vi "TS Calibrate Zero.vi"(8 "error out":errorcluster, 11 "GPIB as string":string="6") -> (0 "error out 2":errorcluster, 3 "GPIB # (out)":string)   [LabVIEW 2015]
uses:
  mc2mc4.llb/MC2/MC4 Wait&ParseSRQ.vi
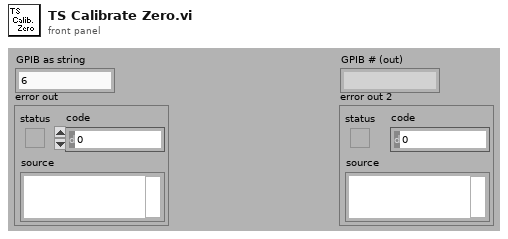
[diagram p1: front panel]
types:
  T1 = enum16{"fine axis move complete", "coarse axis move complete", "either axis move complete", "an axis has reached travel limit"}
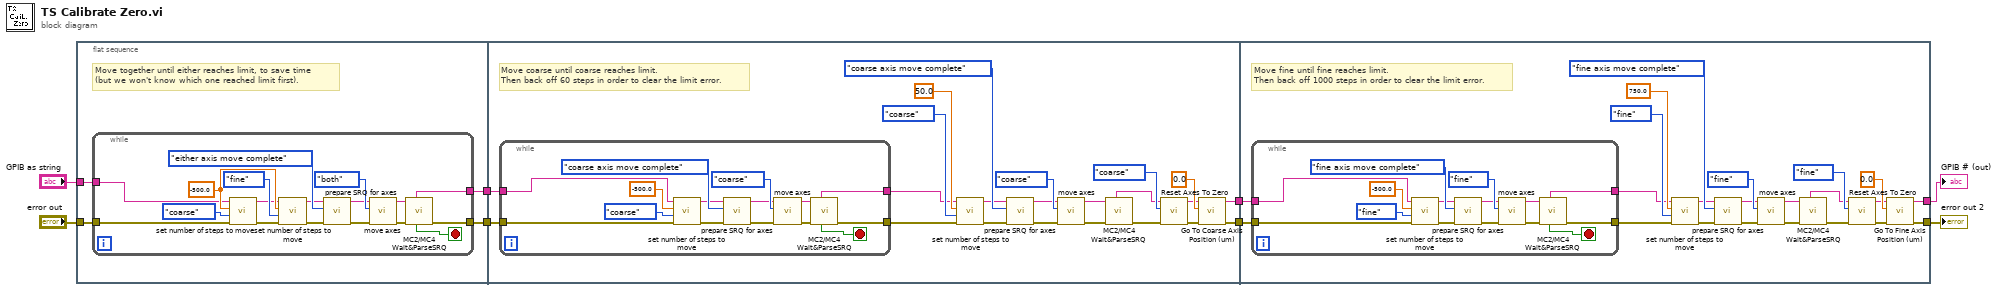
[diagram p0: block diagram]
diagram:
  n1 = flat-sequence {
    tunnel: [w11] -> w8
    tunnel: "error out" -> [w12]
    tunnel: "GPIB as string" -> [w10]
    tunnel: [w9] -> w7
    tunnel: w8 -> [w52]
    tunnel: [w41] -> w6
    tunnel: w7 -> [w38]
    tunnel: [w31] -> w5
    tunnel: w6 -> [w82]
    tunnel: w5 -> [w75]
    tunnel: [w76] -> w1
    tunnel: [w68] -> w2
    frame #0 {
      # "Move together until either reaches limit, to save time\n(but we won't know which one reached limit first)."
      n2 = while {
        tunnel: w12 -> [w13]
        tunnel: [w26] -> w11
        tunnel: w10 -> [w14]
        tunnel: [w15] -> w9
        stop <- w20 stop-if-true
        w24 = -500.0 ("number of steps to set")
        n3 = call "set number of steps to move.vi"("error in"=w13, "axis (def: fine)"=enum16{"fine", "coarse"}."coarse", "number of steps to set"=w24, "GPIB # (in): def. 6"=w14) -> ("error out"=w22:errorcluster, "GPIB # (out)"=w19:string)  [unwired: 6 out]
        n4 = call "set number of steps to move.vi"("error in"=w22, "axis (def: fine)"=enum16{"fine", "coarse"}."fine", "number of steps to set"=w24, "GPIB # (in): def. 6"=w19) -> ("error out"=w21:errorcluster, "GPIB # (out)"=w18:string)  [unwired: 6 out]
        n5 = call "prepare SRQ for axes.vi"("error in (no error)"=w21, "category"=T1."either axis move complete", "GPIB # (in): def. 6"=w18) -> ("error out"=w29:errorcluster, "GPIB # (out):"=w17:string)  [unwired: 7 out]
        n6 = call "move axes.vi"("error in"=w29, "stage to move"=enum16{"both", "fine", "coarse"}."both", "GPIB # (in): def. 6"=w17) -> ("error out"=w28:errorcluster, "GPIB # (out)"=w16:string)  [unwired: 7 out]
        n7 = call "MC2/MC4 Wait&ParseSRQ.vi"("error in (no error)"=w28, "GPIB # (in): def. 6"=w16) -> ("error out"=w26:errorcluster, "Limit_Srq"=w20:bool, "GPIB #(out): def. 6"=w15:string)  [unwired: 7 out]
      }
    }
    frame #1 {
      # "Move coarse until coarse reaches limit.\nThen back off 60 steps in order to clear the limit error."
      n8 = while {
        tunnel: w52 -> [w53]
        tunnel: [w61] -> w42
        tunnel: w38 -> [w54]
        tunnel: [w55] -> w37
        stop <- w59 stop-if-true
        n9 = call "set number of steps to move.vi"("error in"=w53, "axis (def: fine)"=enum16{"fine", "coarse"}."coarse", "number of steps to set"=-500.0, "GPIB # (in): def. 6"=w54) -> ("error out"=w65:errorcluster, "GPIB # (out)"=w58:string)  [unwired: 6 out]
        n10 = call "prepare SRQ for axes.vi"("error in (no error)"=w65, "category"=T1."coarse axis move complete", "GPIB # (in): def. 6"=w58) -> ("error out"=w64:errorcluster, "GPIB # (out):"=w57:string)  [unwired: 7 out]
        n11 = call "move axes.vi"("error in"=w64, "stage to move"=enum16{"both", "fine", "coarse"}."coarse", "GPIB # (in): def. 6"=w57) -> ("error out"=w63:errorcluster, "GPIB # (out)"=w56:string)  [unwired: 7 out]
        n12 = call "MC2/MC4 Wait&ParseSRQ.vi"("error in (no error)"=w63, "GPIB # (in): def. 6"=w56) -> ("error out"=w61:errorcluster, "Limit_Srq"=w59:bool, "GPIB #(out): def. 6"=w55:string)  [unwired: 7 out]
      }
      n13 = call "set number of steps to move.vi"("error in"=w42, "axis (def: fine)"=enum16{"fine", "coarse"}."coarse", "number of steps to set"=50.0, "GPIB # (in): def. 6"=w37) -> ("error out"=w46:errorcluster, "GPIB # (out)"=w36:string)  [unwired: 6 out]
      n14 = call "prepare SRQ for axes.vi"("error in (no error)"=w46, "category"=T1."coarse axis move complete", "GPIB # (in): def. 6"=w36) -> ("error out"=w45:errorcluster, "GPIB # (out):"=w35:string)  [unwired: 7 out]
      n15 = call "move axes.vi"("error in"=w45, "stage to move"=enum16{"both", "fine", "coarse"}."coarse", "GPIB # (in): def. 6"=w35) -> ("error out"=w44:errorcluster, "GPIB # (out)"=w34:string)  [unwired: 7 out]
      n16 = call "MC2/MC4 Wait&ParseSRQ.vi"("error in (no error)"=w44, "GPIB # (in): def. 6"=w34) -> ("error out"=w48:errorcluster, "GPIB #(out): def. 6"=w33:string)  [unwired: 8 out]
      n17 = call "Reset Axes To Zero.vi"("error in"=w48, "axis (def: fine)"=enum16{"both", "fine", "coarse"}."coarse", "GPIB # (in):def. 6"=w33) -> ("error out"=w51:errorcluster, "GPIB # (out)"=w32:string)  [unwired: 7 out]
      n18 = call "Go To Coarse Axis Position (um).vi"("error in (no error)"=w51, "Coarse Axis Position (um)"=dbl[unit] 0.0, "GPIB # (in): def. 6"=w32) -> ("error out"=w41:errorcluster, "GPIB # (out)"=w31:string)  [unwired: 7 out]
    }
    frame #2 {
      # "Move fine until fine reaches limit.\nThen back off 1000 steps in order to clear the limit error."
      n19 = while {
        tunnel: w82 -> [w90]
        tunnel: [w97] -> w81
        tunnel: w75 -> [w91]
        tunnel: [w92] -> w74
        stop <- w96 stop-if-true
        n20 = call "set number of steps to move.vi"("error in"=w90, "axis (def: fine)"=enum16{"fine", "coarse"}."fine", "number of steps to set"=-500.0, "GPIB # (in): def. 6"=w91) -> ("error out"=w100:errorcluster, "GPIB # (out)"=w95:string)  [unwired: 6 out]
        n21 = call "prepare SRQ for axes.vi"("error in (no error)"=w100, "category"=T1."fine axis move complete", "GPIB # (in): def. 6"=w95) -> ("error out"=w101:errorcluster, "GPIB # (out):"=w94:string)  [unwired: 7 out]
        n22 = call "move axes.vi"("error in"=w101, "stage to move"=enum16{"both", "fine", "coarse"}."fine", "GPIB # (in): def. 6"=w94) -> ("error out"=w102:errorcluster, "GPIB # (out)"=w93:string)  [unwired: 7 out]
        n23 = call "MC2/MC4 Wait&ParseSRQ.vi"("error in (no error)"=w102, "GPIB # (in): def. 6"=w93) -> ("error out"=w97:errorcluster, "Limit_Srq"=w96:bool, "GPIB #(out): def. 6"=w92:string)  [unwired: 7 out]
      }
      n24 = call "set number of steps to move.vi"("error in"=w81, "axis (def: fine)"=enum16{"fine", "coarse"}."fine", "number of steps to set"=750.0, "GPIB # (in): def. 6"=w74) -> ("error out"=w86:errorcluster, "GPIB # (out)"=w73:string)  [unwired: 6 out]
      n25 = call "prepare SRQ for axes.vi"("error in (no error)"=w86, "category"=T1."fine axis move complete", "GPIB # (in): def. 6"=w73) -> ("error out"=w87:errorcluster, "GPIB # (out):"=w72:string)  [unwired: 7 out]
      n26 = call "move axes.vi"("error in"=w87, "stage to move"=enum16{"both", "fine", "coarse"}."fine", "GPIB # (in): def. 6"=w72) -> ("error out"=w88:errorcluster, "GPIB # (out)"=w71:string)  [unwired: 7 out]
      n27 = call "MC2/MC4 Wait&ParseSRQ.vi"("error in (no error)"=w88, "GPIB # (in): def. 6"=w71) -> ("error out"=w84:errorcluster, "GPIB #(out): def. 6"=w70:string)  [unwired: 8 out]
      n28 = call "Reset Axes To Zero.vi"("error in"=w84, "axis (def: fine)"=enum16{"both", "fine", "coarse"}."fine", "GPIB # (in):def. 6"=w70) -> ("error out"=w77:errorcluster, "GPIB # (out)"=w69:string)  [unwired: 7 out]
      n29 = call "Go To Fine Axis Position (um).vi"("error in"=w77, "Fine Axis Position (um)"=dbl[unit] 0.0 ("Coarse Axis Position (um)"), "GPIB # (in): def. 6"=w69) -> ("error out"=w76:errorcluster, "GPIB # (out)"=w68:string)  [unwired: 7 out]
    }
  }
  "GPIB # (out)" <- w2
  "error out 2" <- w1
